vi "Write Section Ref.vi"(7 "Section Name":string, 8 "error in (no error)":errorcluster, 10 "Section (Cluster)":variant, 11 "Refnum in":T1) -> (0 "error out":errorcluster, 3 "Refnum out":T1)   [LabVIEW 2024, in "Generic Config Handling.lvlib"]
doc: "This vi writes the cluster as a section in the config file. \n\nIf section name is not wired then the default is to use the name of the cluster.\n\nEach element of the cluster becomes a key, therefore it must be named, and they should be unique and not include any special characters (spaces are allowed and are replaced by_)\n\nYou cannot nest clusters and only simple datatypes are allowed. 1D and 2D arrays are allowed. They are stored as a single element with columns delimited by semicolons and rows delimited by commas. 1D arrays are stored as a single row (ie. comma delimited). \n\nEnums are stored as U32s."
uses:
  Generic Config Handling.lvlib
  <vilib>/Utility/config.llb/Config Data RefNum.ctl
  <vilib>/Utility/VariantDataType/VariantType.lvlib
  <vilib>/Utility/config.llb/NI_LVConfig.lvlib
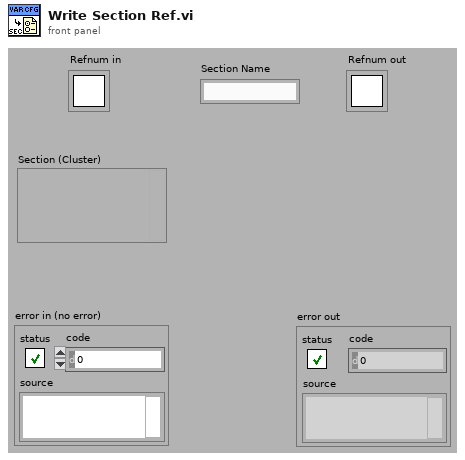
[diagram p1: front panel]
types:
  T1 = typedef "NI_LVConfig.lvlib/Config Data RefNum.ctl" = refnum<k1>
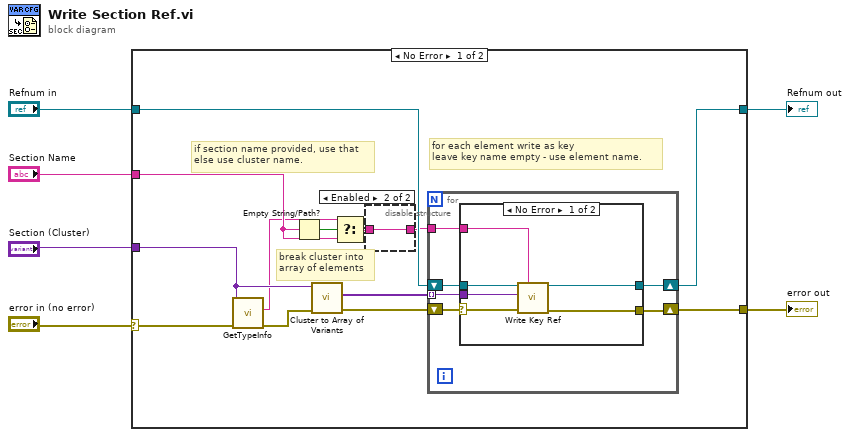
[diagram p0: block diagram]
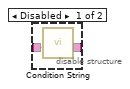
[diagram p2: hidden frame]
diagram:
  n1 = case shown="No Error" "error in (no error)" {
    selector: "error in (no error)" -> [w7 w38]
    tunnel: "Refnum in" -> [w18 w37]
    tunnel: [w17 w37] -> w5
    tunnel: [w16 w38] -> w4
    tunnel: "Section Name" -> [w14 _]
    tunnel: "Section (Cluster)" -> [w11 _]
    frame No Error {
      # "for each element write as key\nleave key name empty - use element name."
      # "break cluster into \narray of elements"
      # "if section name provided, use that\nelse use cluster name."
      n2 = call <vilib>:"GetTypeInfo.vi"("error in (no error)"=w7, "Variant"=w11) -> ("error out"=w9:errorcluster, "Name"=w10:string)  [unwired: 5 in, 3 out]
      n3 = Empty String/Path?(string/path=w14) -> (empty?=w15:bool)
      n4 = call "Cluster to Array of Variants.vi"("error in (no error)"=w9, "Section (Cluster)"=w11) -> ("error out"=w8:errorcluster, "Cluster Elements"=w19:variant[])  [unwired: 7 in, 1 out]
      n5 = Select(t=w10, s=w15, f=w14) -> (s? t:f=w12:string)
      n6 = disable-structure shown="Enabled" {
        disable-tunnel: [w21 w22] -> w13
        disable-tunnel: w12 -> [w20 w22]
        frame Disabled {
          n7 = call "Condition String.vi"("input string"=w20) -> ("result string"=w21:string)  [unwired: 9 in, 1 out]
        }
        frame Enabled {
        }
      }
      n8 = for {
        tunnel: w13 -> [w27]
        tunnel: w19 -> [w28] mode=indexing
        shift-right: [w24] -> w16
        shift-left: w8 -> [w23]
        shift-right: [w25] -> w17
        shift-left: w18 -> [w26]
        n9 = case shown="No Error" w23 {
          selector: w23 -> [w29 w36]
          tunnel: w28 -> [w34 _]
          tunnel: w27 -> [w33 _]
          tunnel: w26 -> [w32 w35]
          tunnel: [w31 w35] -> w25
          tunnel: [w30 w36] -> w24
          frame No Error {
            n10 = call "Write Key Ref.vi"("Section"=w33, "error in (no error)"=w29, "Section Element"=w34, "Refnum in"=w32) -> ("error out"=w30:errorcluster, "Refnum out"=w31:T1)  [unwired: 6 in]
          }
          frame Error {
          }
        }
      }
    }
    frame Error {
    }
  }
  "Refnum out" <- w5
  "error out" <- w4
